vi "Diesel 1.vi"() -> ()   [LabVIEW 2018]
uses:
  <vilib>/OPCUA/controls/NodeIds.ctl
  <vilib>/OPCUA/controls/NodeId.ctl
  <vilib>/OPCUA/controls/Write Variant Request.ctl
  <vilib>/OPCUA/controls/Write Status.ctl
  GlobalVal.vi
  <vilib>/OPCUA/client/Multiple Read Variant.vi
  <vilib>/OPCUA/client/Multiple Write Variant.vi
  <vilib>/OPCUA/NI OPC UA Client.lvlib
panel:
  in  "DS001_kP":dbl
  in  "DS001_tf":dbl
  in  "DS001_Ki":dbl
  in  "DS001_Kp":dbl
  in  "DS001_tp":dbl
  in  "DS001_kf":dbl
  out "DS001_tf":dbl
  out "OPCUA Error Log":errorcluster
  out "OPC Server URL":string
  out "DS001_Ki":dbl
  out "DS001_tP":dbl
  out "DS001_kf":dbl
  out "DS001_kP":dbl
  out "DS001_Kp":dbl
  out "low":bool
  out "DS001_f0, f Chart":cluster{dbl, dbl}(graph)
  out "DS001_P0, P Chart":cluster{dbl, dbl}(graph)
  out "Time Stamp":timestamp
  out "Pmin":dbl(slide) scale=480.0..510.0
  out "Pmax":dbl(slide) scale=480.0..510.0
  out "DS001_GasLevel":dbl(knob) scale=0.0..100.0
  in  "stop":bool
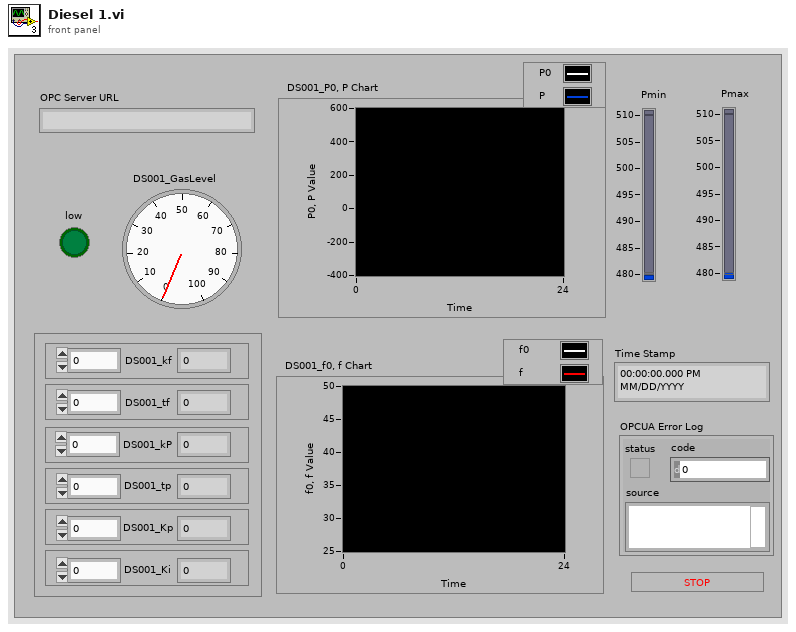
[diagram p1: front panel]
types:
  T1 = typedef "OPC UA Client Refnum.ctl" = refnum<k21>
  T2 = typedef "NodeIds.ctl" = T3[]
  T3 = typedef "NodeId.ctl" = string
  T4 = typedef "Write Variant Request.ctl" = cluster{"node ID":T3, "value":variant, "timestamp (current time)":timestamp, "node status":T5}
  T5 = typedef "Write Status.ctl" = u32
  T6 = typedef "Read Variant Result.ctl" = cluster{"node ID":T3, "value ":variant, "timestamp":timestamp, "status":T7}
  T7 = typedef "OPC UA StatusCode.ctl" = u32
  T8 = cluster{"node ID":T3, "DS001_kP":dbl, "timestamp (current time)":timestamp, "node status":T5}
  T9 = cluster{"node ID":T3, "DS001_tp":dbl, "timestamp (current time)":timestamp, "node status":T5}
  T10 = cluster{"node ID":T3, "DS001_kf":dbl, "timestamp (current time)":timestamp, "node status":T5}
  T11 = cluster{"node ID":T3, "DS001_tf":dbl, "timestamp (current time)":timestamp, "node status":T5}
  T12 = cluster{"node ID":T3, "DS001_Kp":dbl, "timestamp (current time)":timestamp, "node status":T5}
  T13 = cluster{"node ID":T3, "DS001_Ki":dbl, "timestamp (current time)":timestamp, "node status":T5}
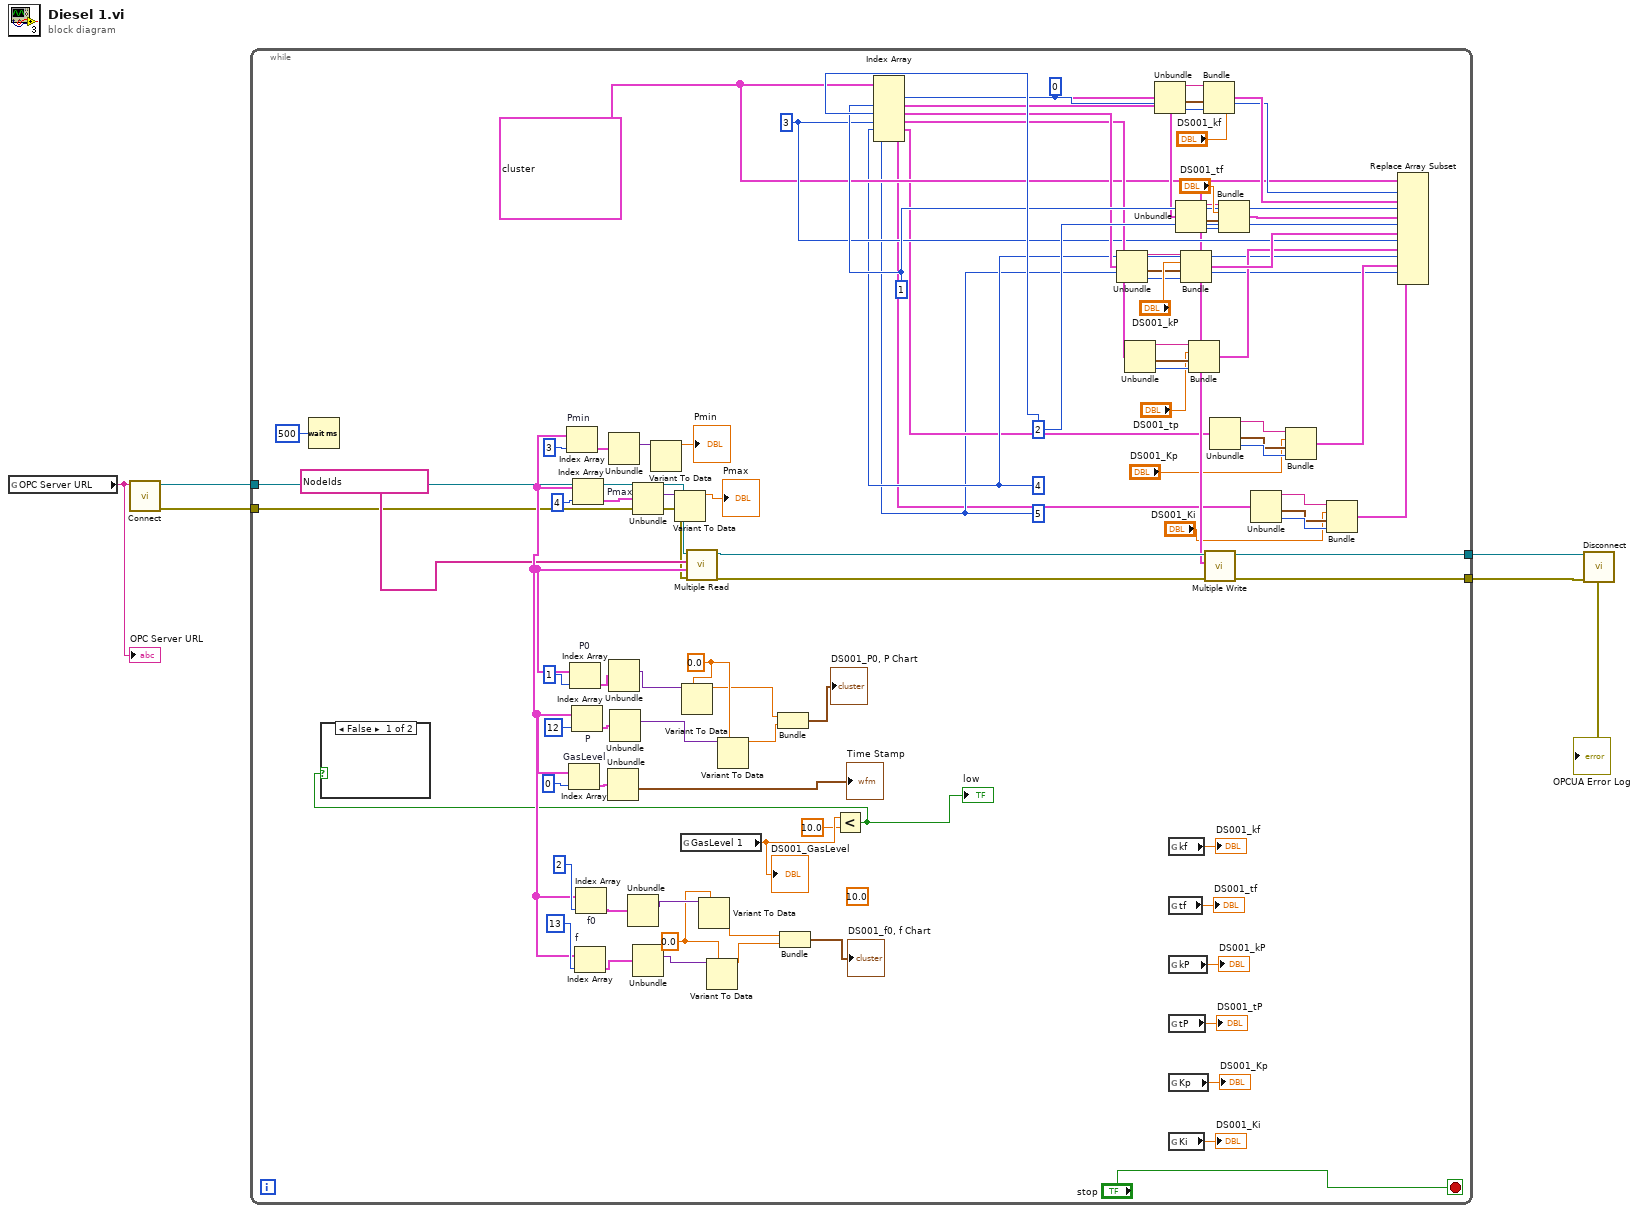
[diagram p0: block diagram]
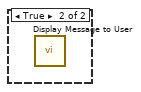
[diagram p2: hidden frame]
diagram:
  n1 = global read "GlobalVal.vi" "OPC Server URL"() -> (w5:string)
  "OPC Server URL" <- w5
  n2 = call <vilib>:"Connect.vi"("server endpoint URL"=w5) -> ("error out"=w2:errorcluster, "OPC UA client refnum out"=w1:T1)  [unwired: 8 in, 1 out]
  n3 = while {
    tunnel: [w25] -> w4
    tunnel: [w24] -> w3
    tunnel: w2 -> [w22]
    tunnel: w1 -> [w21]
    stop <- "stop" stop-if-true
    w29 = T4[] [{"node ID"="ns=2;i=8", "value"=variant(dbl 0.0), "timestamp (current time)"=timestamp(0 s since 1904-01-01), "node status"=0}, {"node ID"="ns=2;i=9", "value"=variant(dbl 0.0), "timestamp (current time)"=timestamp(0 s since 1904-01-01), "node status"=0}, {"node ID"="ns=2;i=10", "value"=variant(dbl 0.0), "timestamp (current time)"=timestamp(0 s since 1904-01-01), "node status"=0}, {"node ID"="ns=2;i=11", "value"=variant(dbl 0.0), "timestamp (current time)"=timestamp(0 s since 1904-01-01), "node status"=0}, {"node ID"="ns=2;i=12", "value"=variant(dbl 0.0), "timestamp (current time)"=timestamp(0 s since 1904-01-01), "node status"=0}, {"node ID"="ns=2;i=13", "value"=variant(dbl 0.0), "timestamp (current time)"=timestamp(0 s since 1904-01-01), "node status"=0}] ("requests")
    w8 = 5 ("Index")
    w16 = 4 ("Index")
    w30 = 3 ("Index")
    w49 = 2 ("Index")
    w36 = 1 ("Index")
    w35 = 0 ("Index")
    (unwired) 10.0 ("y")
    w73 = 0.0
    w83 = 0.0
    n4 = Wait (ms)(milliseconds to wait=u32 500) -> ()  [unwired: 1 out]
    n5 = global read "GlobalVal.vi" "GasLevel 1"() -> (w68:dbl)
    "DS001_GasLevel" <- w68
    n6 = call-poly <vilib>:"Multiple Read.vi"("error in (no error)"=w22, "node IDs"=T2 ["ns=2;i=2", "ns=2;i=3", "ns=2;i=4", "ns=2;i=5", "ns=2;i=6", "ns=2;i=7", "ns=2;i=8", "ns=2;i=9", "ns=2;i=10", "ns=2;i=11", "ns=2;i=12", "ns=2;i=13", "ns=2;i=14", "ns=2;i=15"], "OPC UA client refnum in"=w21) -> ("error out"=w26:errorcluster, "results"=w69:T6[], "OPC UA client refnum out"=w27:T1)  [unwired: 5 in, 1 out]
    n7 = Index Array "Pmin"(array=w69, index=3) -> (element=w94:T6)
    n8 = Index Array "GasLevel"(array=w69, index=0) -> (element=w98:T6)
    n9 = Index Array "P0"(array=w69, index=1) -> (element=w96:T6)
    n10 = Index Array "P"(array=w69, index=12) -> (element=w86:T6)
    n11 = Index Array "Pmax"(array=w69, index=4) -> (element=w90:T6)
    n12 = Index Array "f"(array=w69, index=13) -> (element=w75:T6)
    n13 = Index Array "f0"(array=w69, index=2) -> (element=w78:T6)
    n14 = Unbundle(w98) -> ("timestamp"=→"Time Stamp":timestamp)  [unwired: 3 out]
    n15 = Unbundle(w94) -> ("value"=w93:variant)  [unwired: 3 out]
    n16 = Unbundle(w96) -> ("value"=w85:variant)  [unwired: 3 out]
    n17 = Unbundle(w86) -> ("value"=w84:variant)  [unwired: 3 out]
    n18 = Unbundle(w78) -> ("value"=w77:variant)  [unwired: 3 out]
    n19 = Unbundle(w90) -> ("value"=w89:variant)  [unwired: 3 out]
    n20 = Unbundle(w75) -> ("value"=w74:variant)  [unwired: 3 out]
    n21 = Variant To Data(Variant=w93) -> (data=→"Pmin":dbl)  [unwired: 2 in, 1 out]
    n22 = Variant To Data(Variant=w89) -> (data=→"Pmax":dbl)  [unwired: 2 in, 1 out]
    n23 = Variant To Data(type=w83, Variant=w85) -> (data=w80:dbl)  [unwired: 1 in, 1 out]
    n24 = Variant To Data(type=w73, Variant=w77) -> (data=w72:dbl)  [unwired: 1 in, 1 out]
    n25 = Variant To Data(type=w73, Variant=w74) -> (data=w71:dbl)  [unwired: 1 in, 1 out]
    n26 = Variant To Data(type=w83, Variant=w84) -> (data=w81:dbl)  [unwired: 1 in, 1 out]
    n27 = Bundle(w80, w81) -> (→"DS001_P0, P Chart":cluster{dbl, dbl})  [unwired: 1 in]
    n28 = Bundle(w72, w71) -> (→"DS001_f0, f Chart":cluster{dbl, dbl})  [unwired: 1 in]
    n29 = Less?(x=w68, y=10.0) -> (x < y?=w66:bool)
    "low" <- w66
    n30 = case shown="False" w66 {
      frame False {
      }
      frame True {
        n31 = call "Display Message to User"() -> ()  [unwired: 10 in, 2 out]
      }
    }
    n32 = Index Array(array=w29, index #1=w35, index #2=w36, index #3=w49, index #4=w30, index #5=w16, index #6=w8) -> (element #1=w34:T4, element #2=w33:T4, element #3=w32:T4, element #4=w31:T4, element #5=w15:T4, element #6=w7:T4)
    n33 = Unbundle(w32) -> ("node ID"=w52:T3, "timestamp (current time)"=w47:timestamp, "node status"=w48:T5)  [unwired: 1 out]
    n34 = Unbundle(w31) -> ("node ID"=w46:T3, "timestamp (current time)"=w44:timestamp, "node status"=w45:T5)  [unwired: 1 out]
    n35 = Unbundle(w34) -> ("node ID"=w63:T3, "timestamp (current time)"=w62:timestamp, "node status"=w61:T5)  [unwired: 1 out]
    n36 = global read "GlobalVal.vi" "kf"() -> (→"DS001_kf":dbl)
    n37 = global read "GlobalVal.vi" "tf"() -> (→"DS001_tf":dbl)
    n38 = global read "GlobalVal.vi" "kP"() -> (→"DS001_kP":dbl)
    n39 = global read "GlobalVal.vi" "tP"() -> (→"DS001_tP":dbl)
    n40 = global read "GlobalVal.vi" "Kp"() -> (→"DS001_Kp":dbl)
    n41 = global read "GlobalVal.vi" "Ki"() -> (→"DS001_Ki":dbl)
    n42 = Unbundle(w33) -> ("node ID"=w53:T3, "timestamp (current time)"=w57:timestamp, "node status"=w56:T5)  [unwired: 1 out]
    n43 = Bundle("node ID"=w52, "DS001_kP"="DS001_kP", "timestamp (current time)"=w47, "node status"=w48) -> (w50:T8)  [unwired: 1 in]
    n44 = Bundle("node ID"=w46, "DS001_tp"="DS001_tp", "timestamp (current time)"=w44, "node status"=w45) -> (w43:T9)  [unwired: 1 in]
    n45 = Bundle("node ID"=w63, "DS001_kf"="DS001_kf", "timestamp (current time)"=w62, "node status"=w61) -> (w58:T10)  [unwired: 1 in]
    n46 = Unbundle(w15) -> ("node ID"=w20:T3, "timestamp (current time)"=w18:timestamp, "node status"=w19:T5)  [unwired: 1 out]
    n47 = Bundle("node ID"=w53, "DS001_tf"="DS001_tf", "timestamp (current time)"=w57, "node status"=w56) -> (w55:T11)  [unwired: 1 in]
    n48 = Unbundle(w7) -> ("node ID"=w13:T3, "timestamp (current time)"=w11:timestamp, "node status"=w12:T5)  [unwired: 1 out]
    n49 = Bundle("node ID"=w20, "DS001_Kp"="DS001_Kp", "timestamp (current time)"=w18, "node status"=w19) -> (w14:T12)  [unwired: 1 in]
    n50 = Bundle("node ID"=w13, "DS001_Ki"="DS001_Ki", "timestamp (current time)"=w11, "node status"=w12) -> (w9:T13)  [unwired: 1 in]
    n51 = Replace Array Subset(array=w29, new element #1=w58, index #1=w35, new element #2=w55, index #2=w36, new element #3=w50, index #3=w49, new element #4=w43, index #4=w30, new element #5=w14, index #5=w16, new element #6=w9, index #6=w8) -> (w23:T4[])
    n52 = call-poly <vilib>:"Multiple Write.vi"("error in (no error)"=w26, "requests"=w23, "OPC UA client refnum in"=w27) -> ("error out"=w25:errorcluster, "OPC UA client refnum out"=w24:T1)  [unwired: 5 in, 2 out]
  }
  n53 = call <vilib>:"Disconnect.vi"("error in (no error)"=w4, "OPC UA client refnum in"=w3) -> ("error out"=→"OPCUA Error Log":errorcluster)  [unwired: 9 in]
